vi "F Dwf Digital Can Tx.vi"(5 "rgTX":string, 6 "cDLC":i32, 7 "fRemote":i32, 8 "error in (no error)":errorcluster, 9 "fExtended":i32, 10 "vID":i32, 11 "hdwf":i32) -> (0 "error out":errorcluster, 2 "function return":i32, 3 "rgTX out":string)   [LabVIEW 2019, in "Olasdwf.lvlib"]
doc: "DWFAPI int FDwfDigitalCanTx(HDWF hdwf, int vID, int fExtended, int fRemote, int cDLC, unsigned char *rgTX);"
uses:
  Olasdwf.lvlib
  Windows/System32/dwf.dll
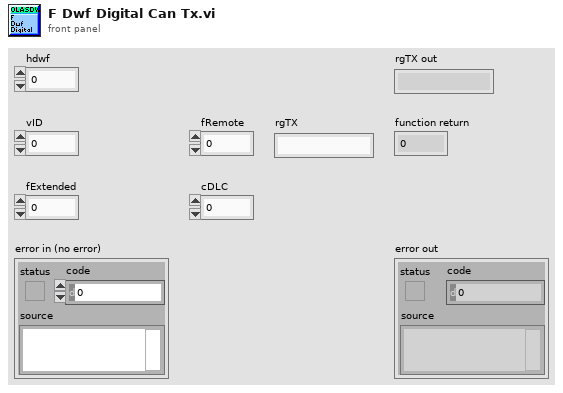
[diagram p1: front panel]
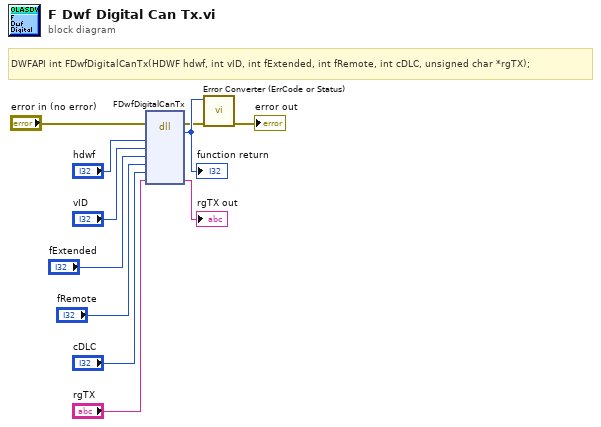
[diagram p0: block diagram]
diagram:
  # "DWFAPI int FDwfDigitalCanTx(HDWF hdwf, int vID, int fExtended, int fRemote, int cDLC, unsigned char *rgTX);"
  n1 = dll-call lib="C:/Windows/System32/dwf.*" fn="FDwfDigitalCanTx"(error in="error in (no error)", "hdwf"="hdwf", "vID"="vID", "fExtended"="fExtended", "fRemote"="fRemote", "cDLC"="cDLC", "rgTX"="rgTX") -> (error out=w2:errorcluster, w11:i32, "rgTX"=→"rgTX out":string)  [unwired: 7 in, 1 out]
  "function return" <- w11
  n2 = call "Error Converter (ErrCode or Status).vi"("error in (no error)"=w2, "error code"=w11) -> ("error out"=→"error out":errorcluster)  [unwired: 9 in]
